vi "To String.vi"(8 "error in (no error)":errorcluster, 11 "String Result in":refnum<class "String Result.lvclass">) -> (0 "error out":errorcluster, 2 "String":string, 3 "String Result out":refnum<class "String Result.lvclass">)   [LabVIEW 2024, in "String Result.lvclass"]
uses:
  String Result.lvclass
  String Result.lvclass/String Result.ctl
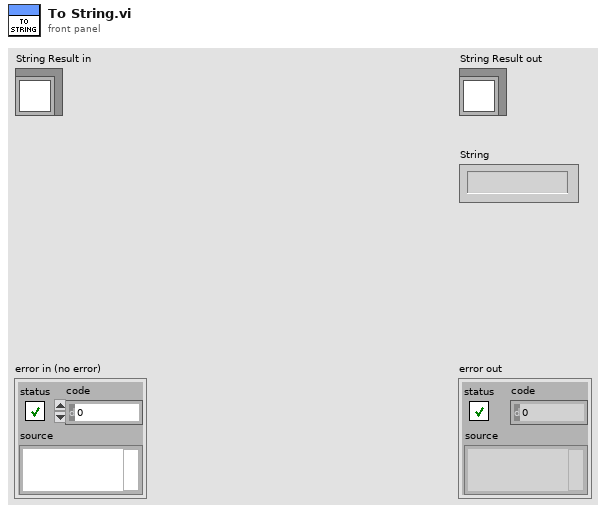
[diagram p1: front panel]
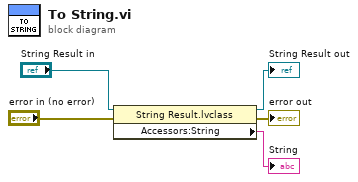
[diagram p0: block diagram]
diagram:
  n1 = property class="String Result.lvclass"(reference="String Result in", error in="error in (no error)") -> (reference out=→"String Result out":refnum<class "String Result.lvclass">, error out=→"error out":errorcluster, "Accessors:String"=→"String":string)
